vi "AlliGator Hot Pixel Removal Options String.vi"(8 "error in (no error)":errorcluster, 11 "Image Display Options":T1 {"Percentile" min=0 max=100}) -> (0 "error out":errorcluster, 3 "String out":string)   [LabVIEW 2021, in "AlliGator Settings.lvlib"]
doc: "Builds a string defining the hot pixel removal options."
uses:
  AlliGator Settings.lvlib
  SwissSPAD/SwissSPAD Live_Image Display Options.ctl
  SwissSPAD/SwissSPAD Live.lvlib
panel:
  # "see the AlliGator License on the block diagram (Ctrl+E or Window:Show Block Diagram)"
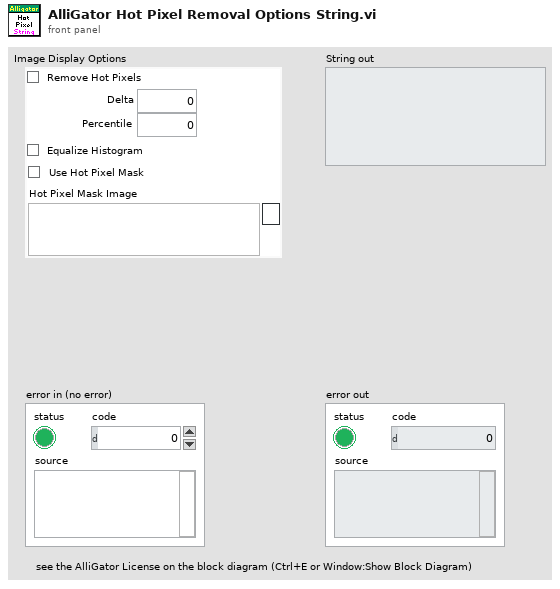
[diagram p1: front panel]
types:
  T1 = typedef "SwissSPAD Live.lvlib/SwissSPAD Live_Image Display Options.ctl" = cluster{"Remove Screamers":bool, "Delta":sgl, "Equalize Histogram":bool, "Percentile":sgl, "Hot Pixel Mask Image":path, "Use Hot Pixel Mask":bool}
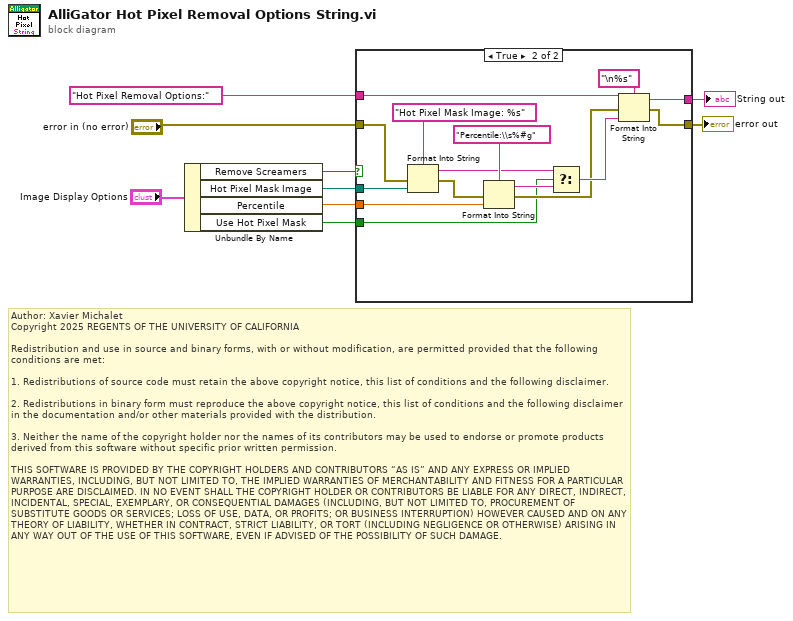
[diagram p0: block diagram]
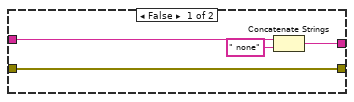
[diagram p2: hidden frame]
diagram:
  # "Author: Xavier Michalet\nCopyright 2025 REGENTS OF THE UNIVERSITY OF CALIFORNIA\n\nRedistribution and use in source and binary forms, with or without modification, are permitted provided that the following conditions are met:\n\n1. Redistributions of source code must retain the above copyright notice, this list of conditions and the following disclaimer.\n\n2. Redistributions in binary form must reproduce the above copyright notice, this list of conditions and the following disclaimer in the documentation and/or other materials provided with the distribution.\n\n3. Neither the name of the copyright holder nor the names of its contributors may be used to endorse or promote products derived from this software without specific prior written permission.\n\nTHIS SOFTWARE IS PROVIDED BY THE COPYRIGHT HOLDERS AND CONTRIBUTORS “AS IS” AND ANY EXPRESS OR IMPLIED WARRANTIES, INCLUDING, BUT NOT LIMITED TO, THE IMPLIED WARRANTIES OF MERCHANTABILITY AND FITNESS FOR A PARTICULAR PURPOSE ARE DISCLAIMED. IN NO EVENT SHALL THE COPYRIGHT HOLDER OR CONTRIBUTORS BE LIABLE FOR ANY DIRECT, INDIRECT, INCIDENTAL, SPECIAL, EXEMPLARY, OR CONSEQUENTIAL DAMAGES (INCLUDING, BUT NOT LIMITED TO, PROCUREMENT OF SUBSTITUTE GOODS OR SERVICES; LOSS OF USE, DATA, OR PROFITS; OR BUSINESS INTERRUPTION) HOWEVER CAUSED AND ON ANY THEORY OF LIABILITY, WHETHER IN CONTRACT, STRICT LIABILITY, OR TORT (INCLUDING NEGLIGENCE OR OTHERWISE) ARISING IN ANY WAY OUT OF THE USE OF THIS SOFTWARE, EVEN IF ADVISED OF THE POSSIBILITY OF SUCH DAMAGE."
  n1 = Unbundle By Name("Image Display Options") -> ("Remove Screamers"=w8:bool, "Hot Pixel Mask Image"=w3:path, "Percentile"=w2:sgl, "Use Hot Pixel Mask"=w1:bool)
  n2 = case shown="True" w8 {
    tunnel: "error in (no error)" -> [w10 w16]
    tunnel: [w10 w28] -> w6
    tunnel: [w12 w27] -> w5
    tunnel: "Hot Pixel Removal Options:" ("initial string") -> [w13 w25]
    tunnel: w3 -> [_ w23]
    tunnel: w2 -> [_ w21]
    tunnel: w1 -> [_ w14]
    frame False {
      n3 = Concatenate Strings(w13, " none" ("string")) -> (w12:string)
    }
    frame True {
      n4 = Format Into String(format string="Hot Pixel Mask Image: %s", error in=w16, w23) -> (resulting string=w20:string, error out=w17:errorcluster)  [unwired: 1 in]
      n5 = Format Into String(format string="Percentile:\\s%#g", error in=w17, w21) -> (resulting string=w19:string, error out=w15:errorcluster)  [unwired: 1 in]
      n6 = Select(t=w20, s=w14, f=w19) -> (s? t:f=w18:string)
      n7 = Format Into String(format string="\n%s", initial string=w25, error in=w15, w18) -> (resulting string=w27:string, error out=w28:errorcluster)
    }
  }
  "error out" <- w6
  "String out" <- w5
